vi "U3 Stream Example LJ_swNONE.vi"() -> ()   [LabVIEW 2021]
panel:
  in  "Resolution Index":u8
  out "Waveform Graph":dbl[][](graph)
  out "# Skipped Scans":i32
  in  "Simulated Processing Delay [ms]":u32
  out "UD Backlog [%]":dbl format="%.2f"
  in  "Scan List":u8[](array[numeric])=[0, 1, 2, 3]
  out "Actual Scan Rate (Hz)":dbl=1000.0 format="%.3f"
  out "ms Per Loop":u32
  out "U3 Backlog [%]":dbl format="%.2f"
  out "Scans Retrieved Sec (measured)":dbl format="%.2f"
  out "# Scans Read":i32
  out "# of iterations":i32
  out "Data":dbl[][](array[numeric]) format="%.3f"
  in  "Scan Rate (Hz)":dbl=1000.0 format="%.3f"
  in  "Data File Extension":string="dat"
  out "Current Data File":path
  in  "Data File Prefix":string="data"
  in  "Write To File":bool
  in  "FirstFound":bool=TRUE
  in  "stop":bool
  in  "Address":string="1"
  out "Error Message":string
  # "Streams using the NONE wait mode.  Streaming\nrequires U3 hardware revision 1.21."
  # "The actual scans/sec is controlled\nby hardware and is known.  This\n\"measured\" suggests the rate at\nwhich data is being retreived."
  # "0=Auto"
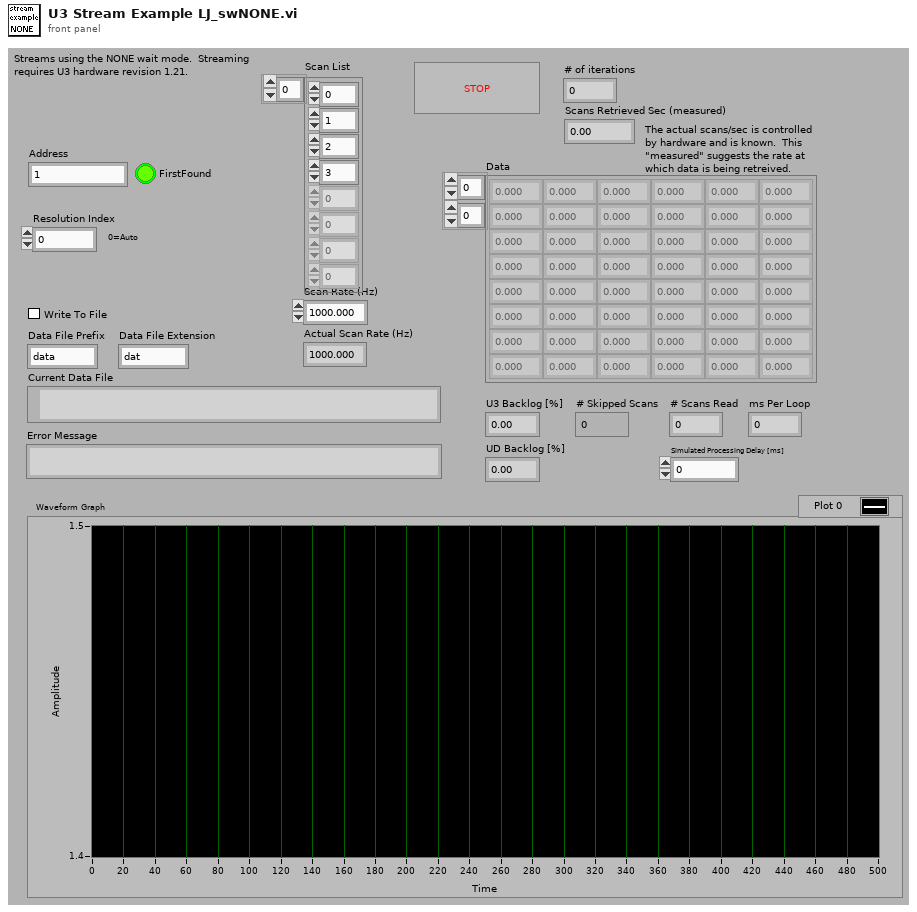
[diagram p1: front panel]
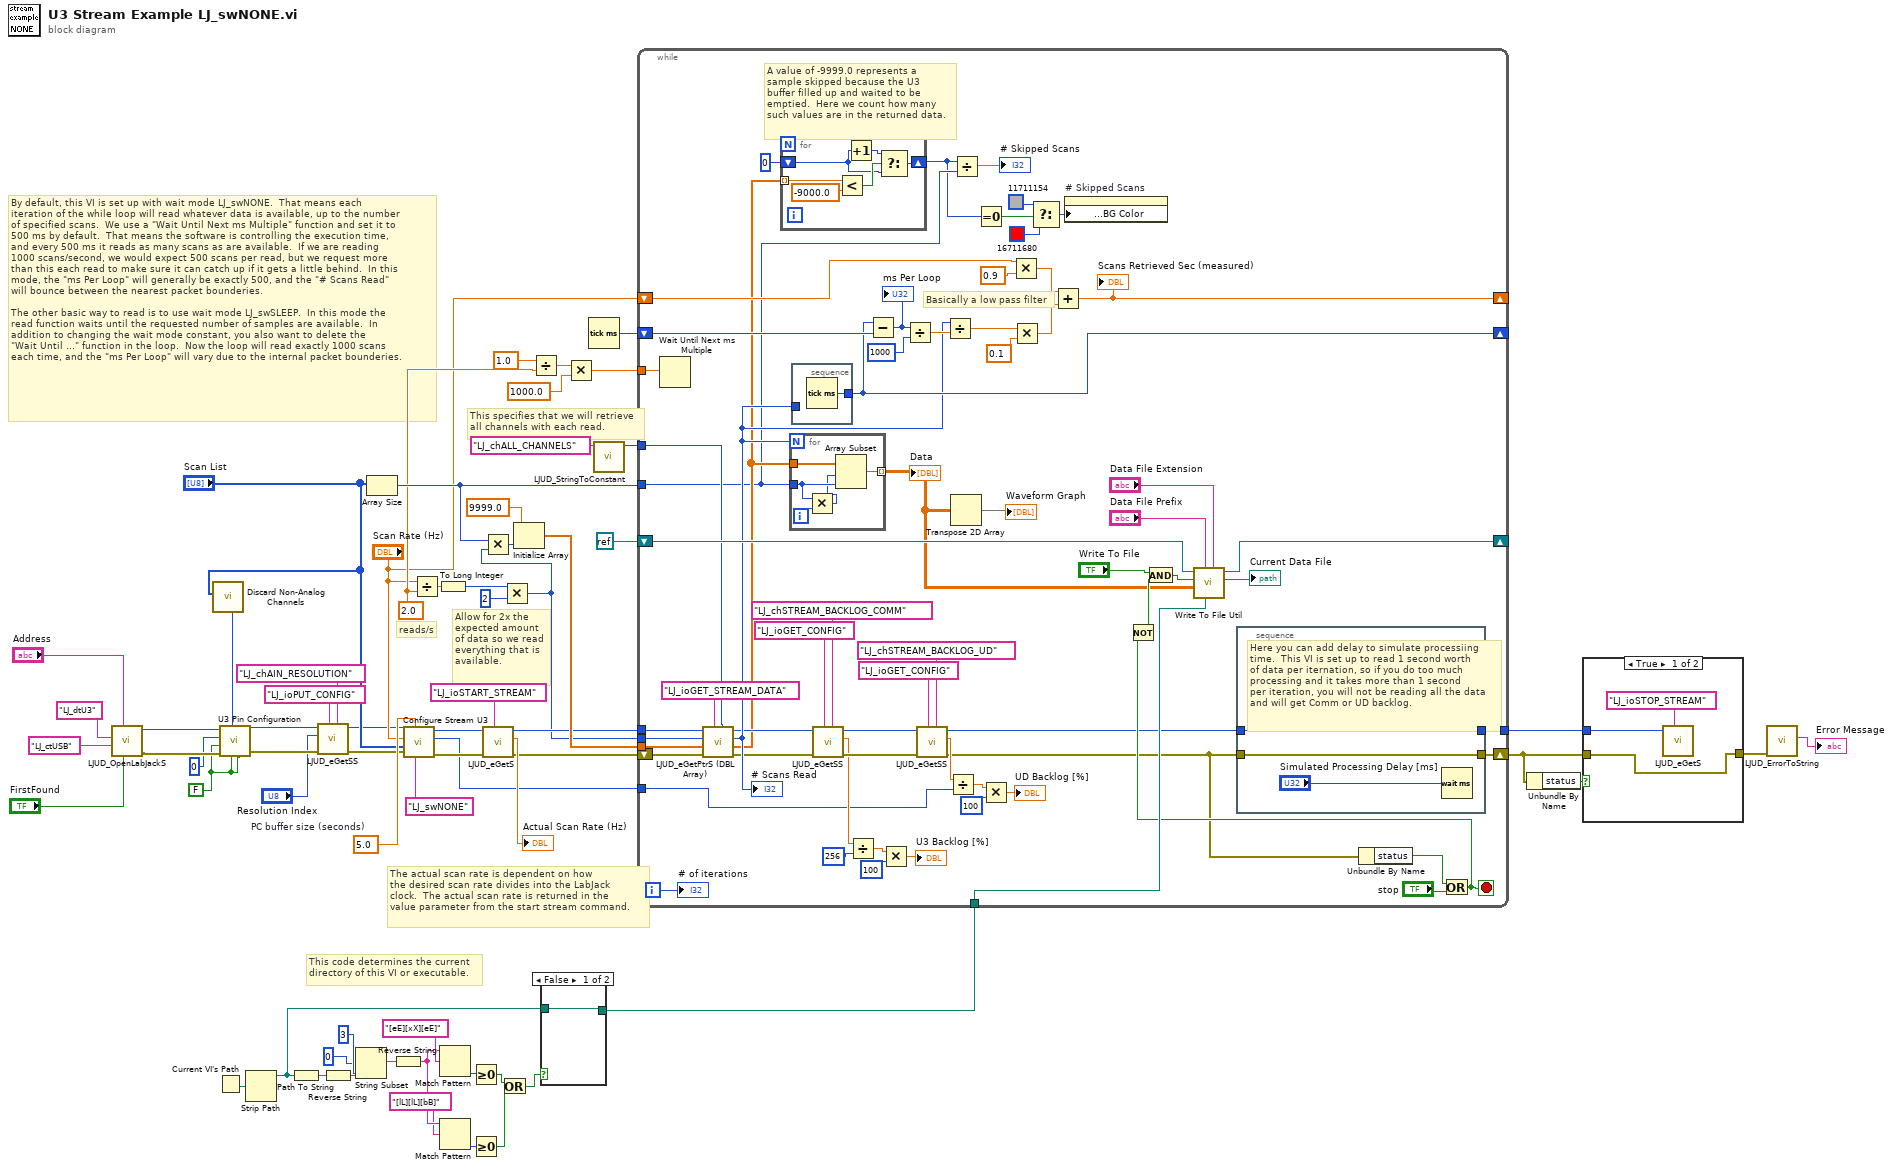
[diagram p0: block diagram]
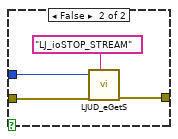
[diagram p2: hidden frame]
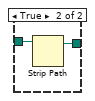
[diagram p3: hidden frame]
diagram:
  w11 = 2.0 ("y")
  w21 = FALSE ("Enable DAC1")
  w34 = 5.0  # PC buffer size (seconds)
  # "reads/s"
  # "Allow for 2x the\nexpected amount\nof data so we read\neverything that is\navailable."
  # "By default, this VI is set up with wait mode LJ_swNONE.  That means each\niteration of the while loop will read whatever data is available, up to the number\nof specified scans.  We use a \"Wait Until Next ms Multiple\" function and set it to\n500 ms by default.  That means the software is controlling the execution time,\nand every 500 ms it reads as many scans as are available.  If we are reading\n1000 scans/second, we would expect 500 scans per read, but we request more\nthan this each read to make sure it can catch up if it gets a little behind.  In this\nmode, the \"ms Per Loop\" will generally be exactly 500, and the \"# Scans Read\"\nwill bounce between the nearest packet bounderies.\n\nThe other basic way to read is to use wait mode LJ_swSLEEP.  In this mode the\nread function waits until the requested number of samples are available.  In\naddition to changing the wait mode constant, you also want to delete the\n\"Wait Until ...\" function in the loop.  Now the loop will read exactly 1000 scans\neach time, and the \"ms Per Loop\" will vary due to the internal packet bounderies."
  # "This specifies that we will retrieve\nall channels with each read."
  # "The actual scan rate is dependent on how\nthe desired scan rate divides into the LabJack\nclock.  The actual scan rate is returned in the\nvalue parameter from the start stream command."
  # "This code determines the current\ndirectory of this VI or executable."
  n1 = call "LJUD_OpenLabJackS.vi"("FirstFound"="FirstFound", "Address"="Address", "ConnectionType"="LJ_ctUSB", "DeviceType"="LJ_dtU3") -> ("error out"=w24:errorcluster, "Handle"=w25:i32)  [unwired: 5 in, 1 out]
  n2 = call "Discard Non-Analog Channels.vi"("Channels In"="Scan List") -> ("FIO/EIO Analog Enable"=w20:i32)  [unwired: 7 in, 3 out]
  n3 = Current VI's Path() -> (path=w62:path)
  n4 = call "U3 Pin Configuration.vi"("Enable Counter1"=w21, "Enable Counter0"=w21, "FIO/EIO Analog Enable"=w20, "error in"=w24, "Enable DAC1"=w21, "Number of Timers Enabled"=u8 0, "Handle In"=w25) -> ("error out"=w6:errorcluster, "Handle Out"=w5:i32)  [unwired: 3 in]
  n5 = Strip Path(path=w62) -> (stripped path=w54:path)  [unwired: 1 out]
  n6 = Path To String(path=w54) -> (string=w61:string)
  n7 = call "LJUD_eGetSS.vi"("Channel"="LJ_chAIN_RESOLUTION", "IOType"="LJ_ioPUT_CONFIG", "error in"=w6, "Value Write"="Resolution Index", "Handle In"=w5) -> ("error out"=w4:errorcluster, "Handle Out"=w3:i32)  [unwired: 4 in, 1 out]
  n8 = Reverse String(1:w61) -> (0:w60:string)
  n9 = String Subset(string=w60, offset (0)=0, length (rest)=3 ("length")) -> (substring=w57:string)
  n10 = Array Size(array="Scan List") -> (size(s)=w40:i32)
  n11 = Reverse String(1:w57) -> (0:w53:string)
  n12 = call "Configure Stream U3.vi"("Wait Mode"="LJ_swNONE" ("Wait Mode (2)"), "PC buffer size (seconds)"=w34, "error in"=w4, "Scan List (+)"="Scan List", "Scan Rate (Hz)"="Scan Rate (Hz)", "Handle In"=w3) -> ("error out"=w44:errorcluster, "PC buffer size (samples)"=w26:i32, "Handle Out"=w45:i32)  [unwired: 3 in]
  n13 = Divide(x="Scan Rate (Hz)", y=w11) -> (x/y=w14:dbl)
  n14 = To Long Integer(number=w14) -> (32bit integer=w13:i32)
  n15 = Match Pattern(string=w53, regular expression="[eE][xX][eE]") -> (offset past match=w55:i32)  [unwired: 1 in, 3 out]
  n16 = Match Pattern(string=w53, regular expression="[lL][lL][bB]") -> (offset past match=w50:i32)  [unwired: 1 in, 3 out]
  n17 = Greater Or Equal To 0?(x=w55) -> (x >= 0?=w51:bool)
  n18 = Greater Or Equal To 0?(x=w50) -> (x >= 0?=w49:bool)
  n19 = call "LJUD_eGetS.vi"("IOType"="LJ_ioSTART_STREAM", "error in"=w44, "Handle In"=w45) -> ("error out"=w28:errorcluster, "Value Read"=→"Actual Scan Rate (Hz)":dbl, "Handle Out"=w32:i32)  [unwired: 6 in]
  n20 = Or(x=w51, y=w49) -> (x .or. y?=w48:bool)
  n21 = Multiply(x=w13, y=2) -> (x*y=w9:i32)
  n22 = Multiply(x=w40, y=w9) -> (x*y=w43:i32)
  n23 = Initialize Array(9999.0, w43) -> (w41:dbl[])
  n24 = Divide(x=1.0, y=w11) -> (x/y=w17:dbl)
  n25 = case shown="False" w48 {
    tunnel: w54 -> [w66 w68]
    tunnel: [w66 w67] -> w47
    frame False {
    }
    frame True {
      n26 = Strip Path(path=w68) -> (stripped path=w67:path)  [unwired: 1 out]
    }
  }
  n27 = Multiply(x=w17, y=1000.0) -> (x*y=w15:dbl)
  n28 = Tick Count (ms)() -> (millisecond timer value=w35:u32)
  n29 = call "LJUD_StringToConstant.vi"("String"="LJ_chALL_CHANNELS") -> ("Constant Number"=w29:i32)  [unwired: 9 in, 1 out]
  n30 = while {
    tunnel: w15 -> [w69]
    tunnel: w26 -> [w87]
    shift-left: w28 -> [w95]
    shift-right: [w83] -> w27
    tunnel: w29 -> [w100]
    shift-left: "Scan Rate (Hz)" -> [w108]
    shift-right: [w105] -> _
    shift-left: w35 -> [w117]
    shift-right: [w114] -> _
    tunnel: [w81] -> w38
    tunnel: w40 -> [w78]
    tunnel: w41 -> [w120]
    tunnel: w9 -> [w119]
    tunnel: w47 -> [w124]
    shift-left: refnum<k0> refnum -> [w130]
    shift-right: [w129] -> _
    tunnel: w32 -> [w122]
    i -> [w118]
    stop <- w123 stop-if-true
    # "A value of -9999.0 represents a\nsample skipped because the U3\nbuffer filled up and waited to be\nemptied.  Here we count how many\nsuch values are in the returned data."
    # "Basically a low pass filter"
    n31 = Wait Until Next ms Multiple(millisecond multiple=w69) -> ()  [unwired: 1 out]
    n32 = call "LJUD_eGetPtrS (DBL Array).vi"("Channel"=w100, "IOType"="LJ_ioGET_STREAM_DATA", "error in"=w95, "DBL Array Write"=w120, "Value"=w119, "Handle In"=w122) -> ("error out"=w103:errorcluster, "DBL Array Read"=w80:dbl[], "Value"=w112:i32, "Handle Out"=w104:i32)  [unwired: 2 in]
    "# Scans Read" <- w112
    n33 = for {
      shift-right: [w135] -> w74
      shift-left: 0 -> [w136]
      tunnel: w80 -> [w139] mode=indexing
      n34 = Less?(x=w139, y=-9000.0) -> (x < y?=w137:bool)
      n35 = Increment(x=w136) -> (x+1=w140:i32)
      n36 = Select(t=w140, s=w137, f=w136) -> (s? t:f=w135:i32)
    }
    n37 = for {
      N: w112 -> [_]
      tunnel: w80 -> [w149]
      tunnel: w78 -> [w148]
      tunnel: [w145] -> w70 mode=indexing
      i -> [w147]
      n38 = Multiply(x=w148, y=w147) -> (x*y=w146:i32)
      n39 = Array Subset(array=w149, index=w146, length=w148) -> (w145:dbl[])
    }
    "Data" <- w70
    n40 = stacked-sequence {
      tunnel: w112 -> [_]
      tunnel: [w144] -> w114
      frame #0 {
        n41 = Tick Count (ms)() -> (millisecond timer value=w144:u32)
      }
    }
    n42 = call "LJUD_eGetSS.vi"("Channel"="LJ_chSTREAM_BACKLOG_COMM", "IOType"="LJ_ioGET_CONFIG", "error in"=w103, "Handle In"=w104) -> ("error out"=w96:errorcluster, "Value Read"=w91:dbl, "Handle Out"=w97:i32)  [unwired: 5 in]
    n43 = Divide(x=w91, y=256) -> (x/y=w94:dbl)
    n44 = Subtract(x=w114, y=w117) -> (x-y=w116:u32)
    "ms Per Loop" <- w116
    n45 = Multiply(x=w94, y=100) -> (x*y=→"U3 Backlog [%]":dbl)
    n46 = Divide(x=w116, y=u32 1000) -> (x/y=w113:dbl)
    n47 = call "LJUD_eGetSS.vi"("Channel"="LJ_chSTREAM_BACKLOG_UD", "IOType"="LJ_ioGET_CONFIG", "error in"=w96, "Handle In"=w97) -> ("error out"=w84:errorcluster, "Value Read"=w86:dbl, "Handle Out"=w82:i32)  [unwired: 5 in]
    n48 = Divide(x=w112, y=w113) -> (x/y=w111:dbl)
    n49 = Divide(x=w86, y=w87) -> (x/y=w88:dbl)
    n50 = Transpose 2D Array(2D array=w70) -> (transposed array=→"Waveform Graph":dbl[][])
    n51 = Divide(x=w74, y=w78) -> (x/y=→"# Skipped Scans":dbl)
    n52 = Equal To 0?(x=w74) -> (x = 0?=w73:bool)
    n53 = Multiply(x=w88, y=100) -> (x*y=→"UD Backlog [%]":dbl)
    n54 = Multiply(x=w108, y=0.9) -> (x*y=w107:dbl)
    n55 = Multiply(x=w111, y=0.1) -> (x*y=w106:dbl)
    n56 = Select(t=u32 11711154, s=w73, f=u32 16711680) -> (s? t:f=w72:u32)
    n57 = Add(x=w107, y=w106) -> (x+y=w105:dbl)
    "Scans Retrieved Sec (measured)" <- w105
    n58 = property on="# Skipped Scans" class="DigNum (strict)"("Numeric Text.Text Colors:BG Color"=w72) -> ()  [unwired: 2 in, 2 out]
    n59 = stacked-sequence {
      tunnel: w84 -> [w143]
      tunnel: [w143] -> w83
      tunnel: w82 -> [w142]
      tunnel: [w142] -> w81
      frame #0 {
        # "Here you can add delay to simulate processiing\ntime.  This VI is set up to read 1 second worth\nof data per iternation, so if you do too much\nprocessing and it takes more than 1 second\nper iteration, you will not be reading all the data\nand will get Comm or UD backlog."
        n60 = Wait (ms)(milliseconds to wait="Simulated Processing Delay [ms]") -> ()  [unwired: 1 out]
      }
    }
    n61 = Unbundle By Name(w84) -> ("status"=w133:bool)
    n62 = Or(x=w133, y="stop") -> (x .or. y?=w123:bool)
    n63 = Not(x=w123) -> (.not. x?=w125:bool)
    n64 = And(x="Write To File", y=w125) -> (x .and. y?=w126:bool)
    n65 = call "Write To File Util.vi"("Data File Extension"="Data File Extension", "Working Directory"=w124, "Data File Prefix"="Data File Prefix", "Data"=w70, "Write To File"=w126, "File Refnum In"=w130) -> ("Current Data File"=→"Current Data File":path, "File Refnum Out"=w129:refnum<file>)  [unwired: 3 in, 1 out]
    "# of iterations" <- w118
  }
  n66 = Unbundle By Name(w27) -> ("status"=w31:bool)
  n67 = case shown="True" w31 {
    tunnel: w38 -> [w151 w155]
    tunnel: [w150 w154] -> w37
    tunnel: w27 -> [w150 w153]
    frame True {
      n68 = call "LJUD_eGetS.vi"("IOType"="LJ_ioSTOP_STREAM", "Handle In"=w151) -> ()  [unwired: 7 in, 3 out]
    }
    frame False {
      n69 = call "LJUD_eGetS.vi"("IOType"="LJ_ioSTOP_STREAM", "error in"=w153, "Handle In"=w155) -> ("error out"=w154:errorcluster)  [unwired: 6 in, 2 out]
    }
  }
  n70 = call "LJUD_ErrorToString.vi"("error in"=w37) -> ("String"=→"Error Message":string)  [unwired: 10 in]
